vi "Plugin Main.vi"(11 "Shared Data from EMA":T2={"Impulse Positions"=[], "Parameter Impuls Series"=[], "Data File"={"Data Channels"=[], "Sample Rate"=0, "Channel List"=[]}, "desacc "={"Threshold 1 [Acc]"=7000.0, "Threshold 2 [% of TH1]"=60, "tolerance"=3, "Search WD "=0.1, " always use TH2"=FALSE, "Range"=2.0, "Max time"=120.0, "Min time"=20.0, "Velocity Threshold"=150}, "Experiment Parameters 2"={"Subject"="", "Strain"="", "Rotation plane"="", "Experimenter"="", "Trial"=0.0, "Time"=0.0}} {"Parameter Impuls Series"."Gain" format="%.1f"; "Parameter Impuls Series"."Offset" format="%.1f"}) -> (3 "Shared Data from EMA 2":T2={"Impulse Positions"=[], "Parameter Impuls Series"=[], "Data File"={"Data Channels"=[], "Sample Rate"=0, "Channel List"=[]}, "desacc "={"Threshold 1 [Acc]"=7000.0, "Threshold 2 [% of TH1]"=60, "tolerance"=3, "Search WD "=0.1, " always use TH2"=FALSE, "Range"=2.0, "Max time"=120.0, "Min time"=20.0, "Velocity Threshold"=150}, "Experiment Parameters 2"={"Subject"="", "Strain"="", "Rotation plane"="", "Experimenter"="", "Trial"=0.0, "Time"=0.0}} {"Parameter Impuls Series"."Gain" format="%.1f"; "Parameter Impuls Series"."Offset" format="%.1f"})   [LabVIEW 2013]
uses:
  Plugin Shared Data.ctl
  core/type-defs/TD_Impulse Parameter.ctl
  res/controls/impuls graph/impuls graph.xctl
  comm/impulse/impulse functions.lvlib
  core/core.lvlib
  plugin data.lvlib
panel:
  out "Impulse Plot":T1(xcontrol)
  in  "Parameter Impuls Series":T3=[{"Color"=4652800, "Visible"=TRUE, "Channel"=5, "Invert"=FALSE, "Desaccade"=FALSE, "Offset"=0.0, "Gain"=1.0}, {"Color"=16860, "Visible"=TRUE, "Channel"=13, "Invert"=FALSE, "Desaccade"=FALSE, "Offset"=0.0, "Gain"=1.0}, {"Color"=16711680, "Visible"=TRUE, "Channel"=21, "Invert"=FALSE, "Desaccade"=FALSE, "Offset"=0.0, "Gain"=1.0}] {"Gain" format="%.1f"; "Offset" format="%.1f"}
  in  "Impulse Direction":bool
  in  "Mean and STD":bool
  in  "Stop Button":bool
  # "Offset         Gain    Inv                    Channel                         Col   Vis   Sac"
  # "Pos"
  # "Neg"
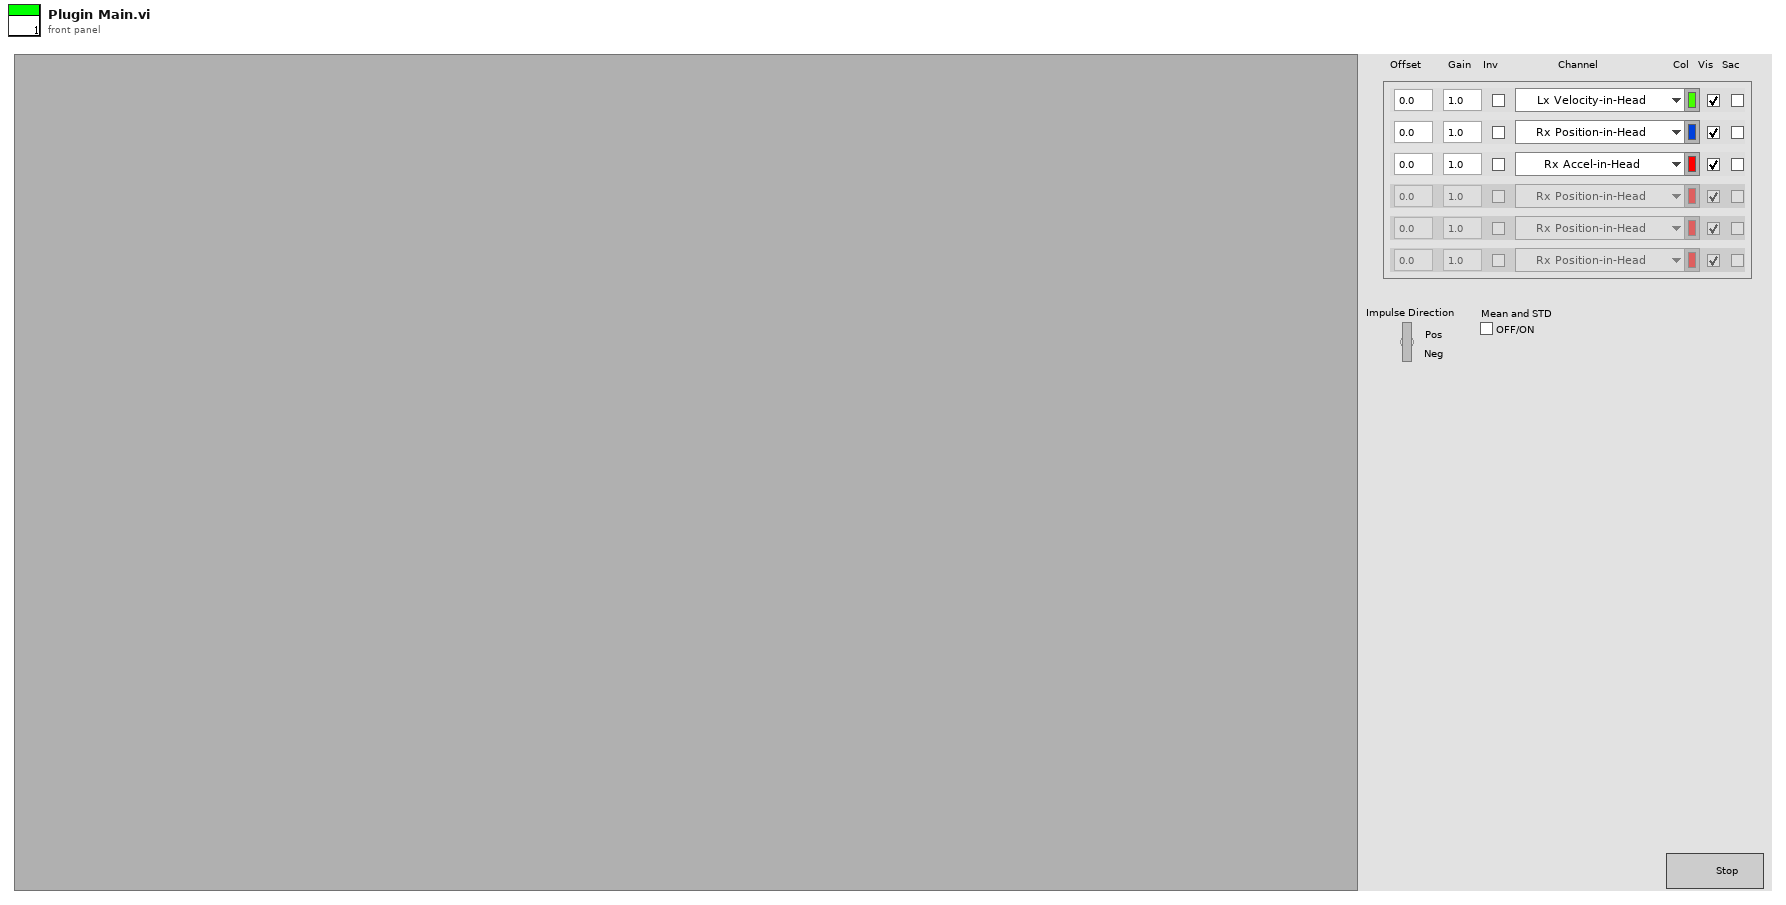
[diagram p1: front panel]
types:
  T1 = cluster{"Data":dbl[][], "Colour":u32, "Channel Name":string, "Sample Rate":dbl, "Visible":bool}[]
  T2 = typedef "plugin data.lvlib/Plugin Shared Data.ctl" = cluster{"Impulse Positions":cluster{"Start":i32, "End":i32, "Impulse Plane":enum16{"Other", "Yaw", "Pitch", "Roll", "LARP", "RALP"}, "Impulse Direction +ve?":bool, "Time offset":i32, "Amplitude offset":dbl}[], "Parameter Impuls Series":T3, "Data File":cluster{"Data Channels":dbl[][], "Sample Rate":i32, "Channel List":string[]}, "desacc ":cluster{"Threshold 1 [Acc]":dbl, "Threshold 2 [% of TH1]":i32, "tolerance":i32, "Search WD ":dbl, " always use TH2":bool, "Range":dbl, "Max time":dbl, "Min time":dbl, "Velocity Threshold":i32}, "Experiment Parameters 2":cluster{"Subject":string, "Strain":string, "Rotation plane":string, "Experimenter":string, "Trial":dbl, "Time":dbl}}
  T3 = typedef "core.lvlib/TD_Impulse Parameter.ctl" = cluster{"Color":u32, "Visible":bool, "Channel":u16, "Invert":bool, "Desaccade":bool, "Offset":dbl, "Gain":dbl}[]
  T4 = enum16{"Other", "Yaw", "Pitch", "Roll", "LARP", "RALP"}
  T5 = cluster{"Data Channels":dbl[][], "Sample Rate":i32, "Channel List":string[]}
  T6 = cluster{"Start":i32, "End":i32, "Impulse Plane":enum16{"Other", "Yaw", "Pitch", "Roll", "LARP", "RALP"}, "Impulse Direction +ve?":bool, "Time offset":i32, "Amplitude offset":dbl}[]
  T7 = cluster{"Threshold 1 [Acc]":dbl, "Threshold 2 [% of TH1]":i32, "tolerance":i32, "Search WD ":dbl, " always use TH2":bool, "Range":dbl, "Max time":dbl, "Min time":dbl, "Velocity Threshold":i32}
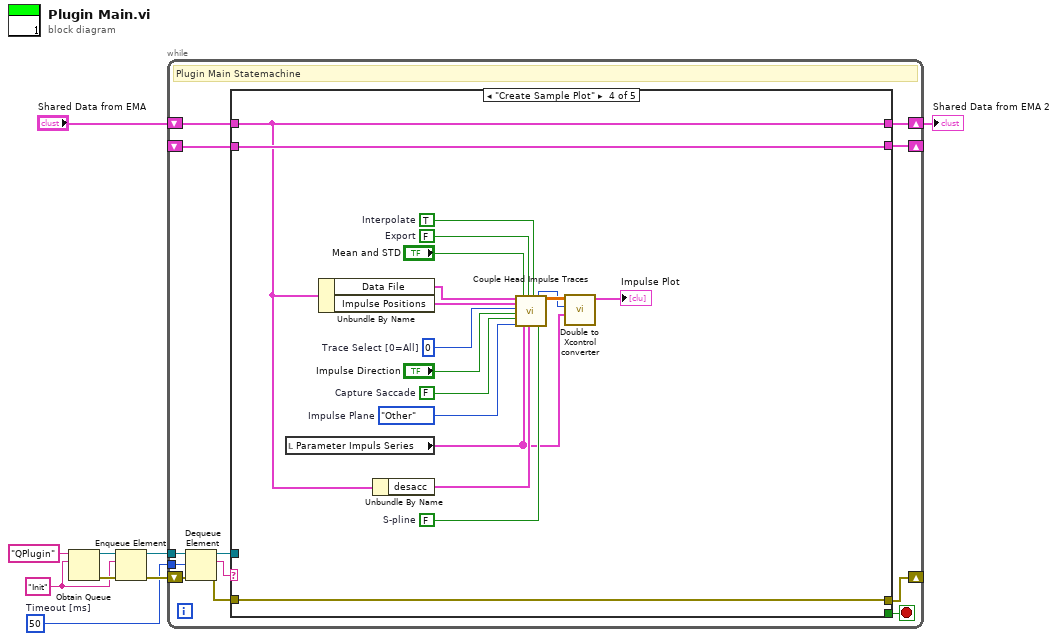
[diagram p0: block diagram]
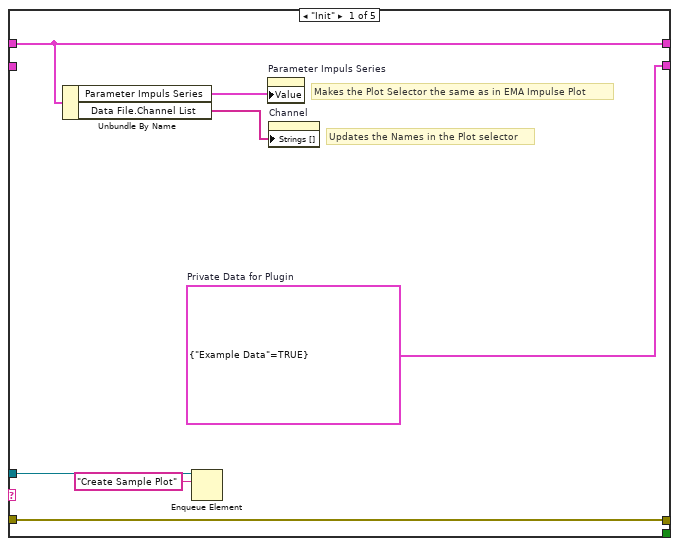
[diagram p2: hidden frame]
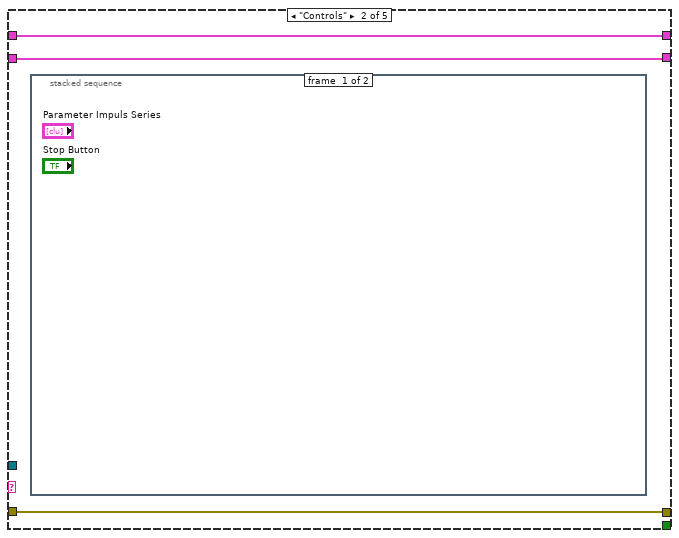
[diagram p3: hidden frame]
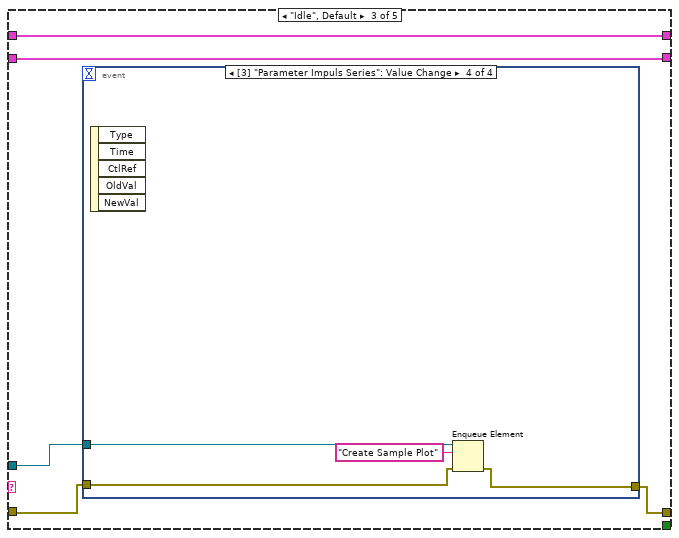
[diagram p5: hidden frame]
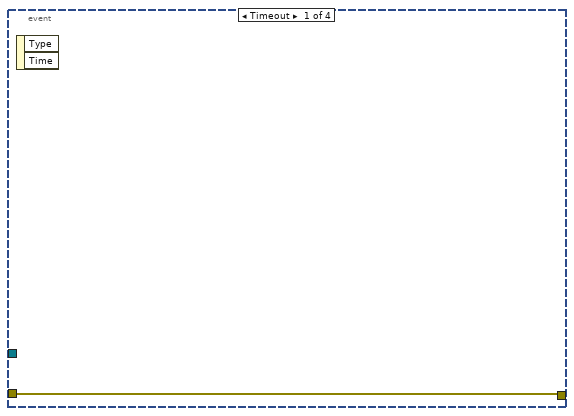
[diagram p6: hidden frame]
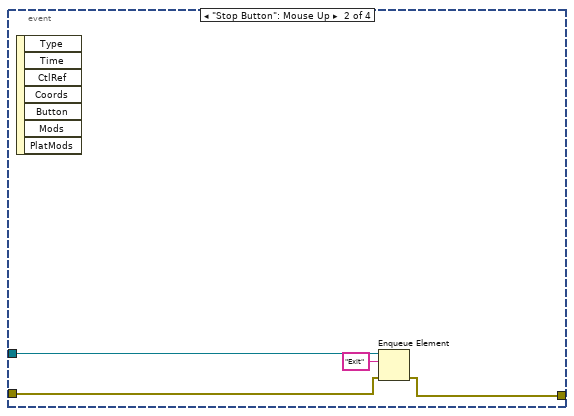
[diagram p7: hidden frame]
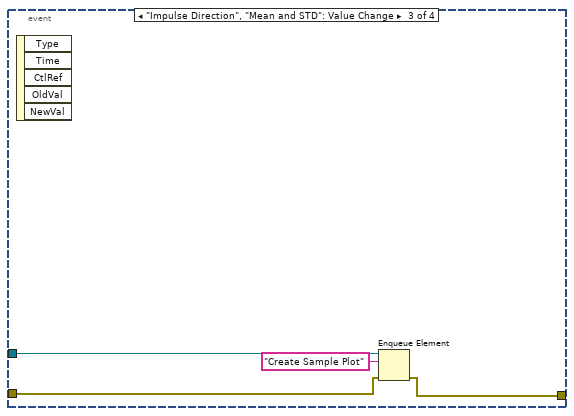
[diagram p8: hidden frame]
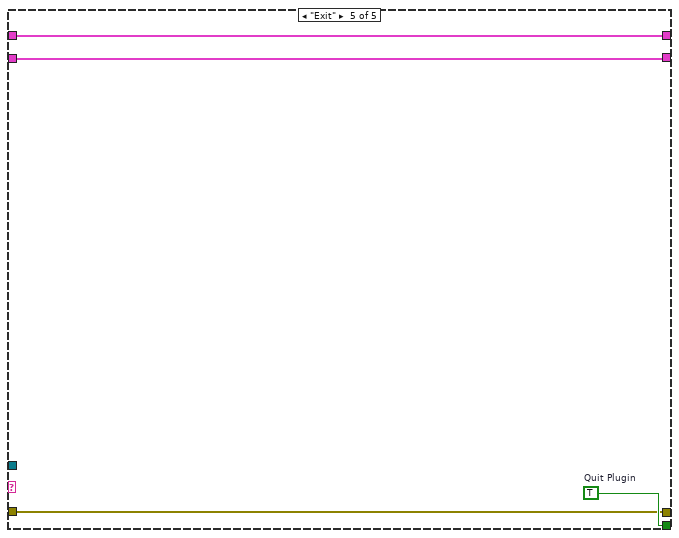
[diagram p9: hidden frame]
diagram:
  w3 = 50  # Timeout [ms]
  w7 = "Init"
  n1 = Obtain Queue(name (unnamed)="QPlugin", element data type=w7) -> (queue out=w8:refnum<queue>, error out=w9:errorcluster)  [unwired: 3 in, 1 out]
  n2 = Enqueue Element(queue=w8, element=w7, error in (no error)=w9) -> (queue out=w5:refnum<queue>, error out=w4:errorcluster)  [unwired: 1 in, 1 out]
  n3 = while {
    tunnel: w5 -> [w20]
    tunnel: w3 -> [w18]
    shift-right: [w14] -> _
    shift-left: w4 -> [w19]
    shift-right: [w13] -> _
    shift-left: _ -> [w12]
    shift-right: [w10] -> w1
    shift-left: "Shared Data from EMA" -> [w11]
    stop <- w21 stop-if-true
    # "Plugin Main Statemachine"
    n4 = Dequeue Element(queue=w20, timeout in ms (-1)=w18, error in (no error)=w19) -> (queue out=w17:refnum<queue>, element=w16:string, error out=w15:errorcluster)  [unwired: 1 out]
    n5 = case shown="\"Create Sample Plot\"" w16 {
      tunnel: [_ _ _ _ w71] -> w21
      tunnel: w17 -> [w26 _ w34 _ _]
      tunnel: w15 -> [w27 w29 w33 w66 w70]
      tunnel: [w27 w29 w32 w66 w70] -> w14
      tunnel: [w28 w30 w36 w67 w69] -> w13
      tunnel: w12 -> [_ w30 w36 w67 w69]
      tunnel: w11 -> [w24 w31 w35 w56 w68]
      tunnel: [w24 w31 w35 w56 w68] -> w10
      frame "Init" {
        w28 = cluster{"Example Data":bool} {"Example Data"=TRUE}  # Private Data for Plugin
        # "Makes the Plot Selector the same as in EMA Impulse Plot"
        # "Updates the Names in the Plot selector"
        n6 = Unbundle By Name(w24) -> ("Parameter Impuls Series"=w23:T3, "Data File.Channel List"=w22:string[])
        n7 = Enqueue Element(queue=w26, element="Create Sample Plot") -> ()  [unwired: 2 in, 3 out]
        n8 = property on="Parameter Impuls Series" class="Arr (strict)"("Value"=w23) -> ()  [unwired: 2 in, 2 out]
        n9 = property on="Channel" class="Ring (strict)"("Strings []"=w22) -> ()  [unwired: 2 in, 2 out]
      }
      frame "Controls" {
        n10 = stacked-sequence {
          frame #0 {
          }
          frame #1 {
          }
        }
      }
      frame "Idle", Default {
        n11 = event shown="[3] \"Parameter Impuls Series\": Value Change" {
          selector: _ -> [_ _ _ _]
          dyn-events: _ -> [_ _ _ _]
          timeout: _ -> [_ _ _ _]
          tunnel: w34 -> [_ w41 w45 w49]
          tunnel: w33 -> [w37 w39 w43 w47]
          tunnel: [w37 w38 w42 w46] -> w32
          event Timeout {
            n12 = event-data() -> ()  [unwired: 1 in, 2 out]
          }
          event "Stop Button": Mouse Up {
            n13 = event-data() -> ()  [unwired: 1 in, 7 out]
            n14 = Enqueue Element(queue=w41, element="Exit", error in (no error)=w39) -> (error out=w38:errorcluster)  [unwired: 1 in, 2 out]
          }
          event "Impulse Direction", "Mean and STD": Value Change {
            n15 = event-data() -> ()  [unwired: 1 in, 5 out]
            n16 = Enqueue Element(queue=w45, element="Create Sample Plot", error in (no error)=w43) -> (error out=w42:errorcluster)  [unwired: 1 in, 2 out]
          }
          event Value Change {
            n17 = event-data() -> ()  [unwired: 1 in, 5 out]
            n18 = Enqueue Element(queue=w49, element="Create Sample Plot", error in (no error)=w47) -> (error out=w46:errorcluster)  [unwired: 1 in, 2 out]
          }
        }
      }
      frame "Create Sample Plot" {
        w54 = FALSE  # S-pline
        w57 = TRUE  # Interpolate
        w58 = FALSE  # Export
        w60 = T4."Other"  # Impulse Plane
        w61 = FALSE  # Capture Saccade
        w63 = 0  # Trace Select [0=All]
        n19 = local read "Parameter Impuls Series"() -> (w51:T3)
        n20 = Unbundle By Name(w56) -> ("Data File"=w64:T5, "Impulse Positions"=w65:T6)
        n21 = Unbundle By Name(w56) -> ("desacc"=w55:T7)
        n22 = call "Couple Head Impulse Traces.vi"("Data Input"=w64, "Impulse Positions"=w65, "Trace Select"=w63, "Impulse Direction +ve?"="Impulse Direction", "Capture Saccade"=w61, "Impulse Plane"=w60, "Mean and STD"="Mean and STD", "Plot Selection 2"=w51, "Export"=w58, "desacc"=w55, "Interpolate"=w57, "S-pline"=w54) -> ("No Impulses"=w52:i32, "Impulses"=w53:dbl[][])  [unwired: 4 in, 2 out]
        n23 = call "Double to Xcontrol converter.vi"("Parameter Impuls Series"=w51, "No Impulses"=w52, "Impulses"=w53) -> ("Array"=→"Impulse Plot":T1)  [unwired: 8 in]
      }
      frame "Exit" {
        w71 = TRUE  # Quit Plugin
      }
    }
  }
  "Shared Data from EMA 2" <- w1
